vi "Send_Pulse.vi"(7 "Filename (.ini)":string="Config_Ver_1\\pulse_sequence.ini", 8 "error in":errorcluster, 11 "VISA arduino in":refnum<visa-resource-name>) -> (0 "error out":errorcluster, 2 "Pulse sequence":T1[](array[typedef]) {"channel" min=2 max=13 step=1}, 3 "VISA arduino out":refnum<visa-resource-name>)   [LabVIEW 2021]
uses:
  Drivers/Arduino_Pulse_Generator/Configurate/Channel_Pulse_Stream.ctl
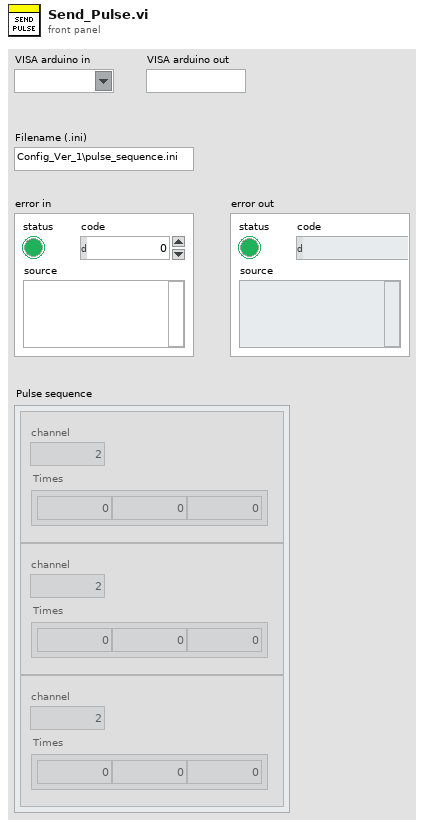
[diagram p1: front panel]
types:
  T1 = typedef "Channel_Pulse_Stream.ctl" = cluster{"Times":dbl[], "channel":u8}
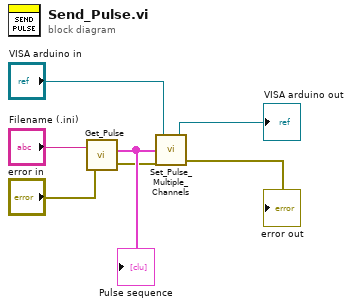
[diagram p0: block diagram]
diagram:
  n1 = call "Get_Pulse.vi"("error in"="error in", "Filename (.ini)"="Filename (.ini)") -> ("error out"=w6:errorcluster, "Pulse sequence"=w7:T1[])
  "Pulse sequence" <- w7
  n2 = call "Set_Pulse_Multiple_Channels.vi"("error in"=w6, "Pulses"=w7, "VISA arduino in"="VISA arduino in") -> ("error out"=→"error out":errorcluster, "VISA arduino out"=→"VISA arduino out":refnum<visa-resource-name>)  [unwired: 1 in]
